vi "Read.vi"(8 "error in (no error)":errorcluster, 11 "CIFTag in":refnum<class "CIFTagI64.lvclass">) -> (0 "error out":errorcluster, 1 "timed out?":bool, 2 "Data":i64, 3 "CIFTag out":refnum<class "CIFTagI64.lvclass">)   [LabVIEW 2021, in "CIFTagI64.lvclass"]
uses:
  CIFTagI64.lvclass
  D:/dev/CIF-LVCore/src/CIFUtilities/CIFChannels/CIFChannels.lvclass
  D:/dev/CIF-LVCore/src/Channels/CIFTag/CIFTag/CIFTag.lvclass
  CIFUtilities/CIFChannels/CIFChannels.lvclass/CIFChannels.ctl
  CIFUtilities/CIFChannels/Typedef/Channel State.ctl
  CIFUtilities/CIFChannels/Typedef/Direction.ctl
  CIFTagI64.lvclass/CIFTagI64.ctl
  CIFTag/CIFTag.lvclass/CIFTag.ctl
  cbead010-ab61-49ec-ac6c-083511305d37.vi
  CIFUtilities/CIFChannels/Accessors/Read Channel State.vi
  CIFUtilities/CIFChannels/Accessors/Read Direction.vi
  CIFUtilities/CIFChannels/Accessors/Write Channel State.vi
  CIFUtilities/CIFChannels/Accessors/Read Disconnect Behavior.vi
  cbead010-ab61-49ec-ac6c-083511305d37.vi/c28b0ead-42ad-4072-80a2-aca7f2bd7ce3.vi
  cbead010-ab61-49ec-ac6c-083511305d37.vi/219d0231-d98b-4193-b5cc-84f90e3c9091.vi
  <vilib>/CIFChannels/SubVIs/Get dll Path.vi
  CIFTag/CIFTag.lvclass
  CIFUtilities/CIFChannels/CIFChannels.lvclass
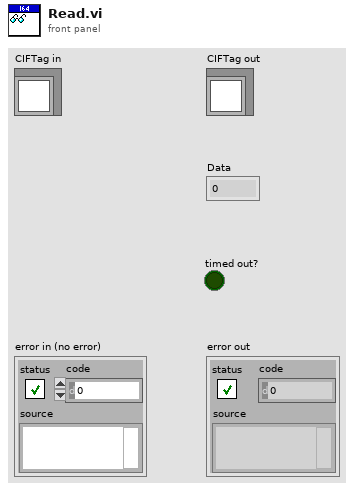
[diagram p1: front panel]
types:
  T1 = typedef "CIFChannels.lvclass/Channel State.ctl" = enum16{"Creating", "Disconnected", "Connecting", "Connected", "Destroying"}
  T2 = typedef "CIFChannels.lvclass/Direction.ctl" = enum16{"Publisher", "Subscriber"}
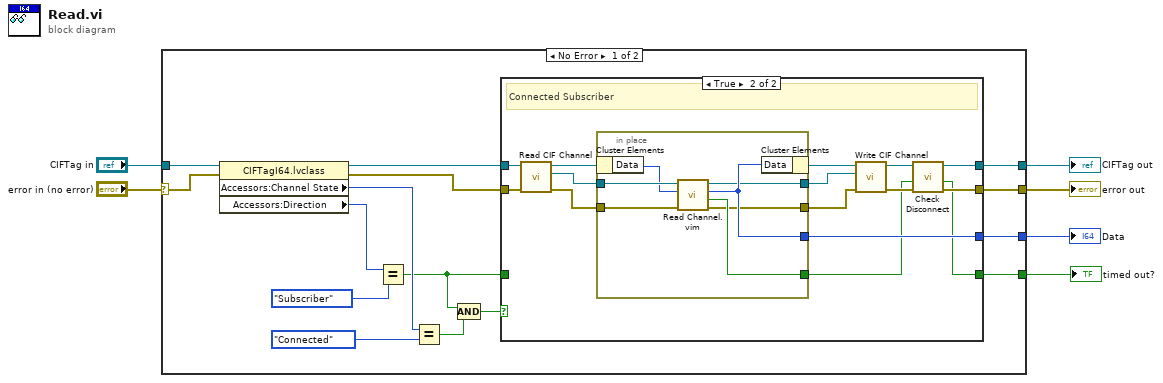
[diagram p0: block diagram]
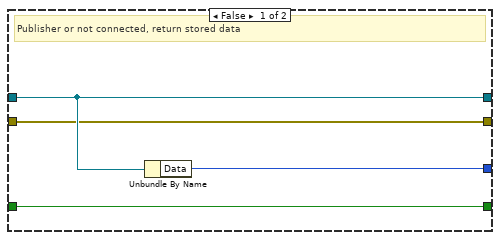
[diagram p2: hidden frame]
diagram:
  n1 = case shown="No Error" "error in (no error)" {
    selector: "error in (no error)" -> [w18 w49]
    tunnel: [w7 w49] -> w5
    tunnel: [w8 w48] -> w3
    tunnel: "CIFTag in" -> [w19 w48]
    tunnel: [w21 _] -> w2
    tunnel: [w20 _] -> w1
    frame No Error {
      n2 = property class="CIFTagI64.lvclass"(reference=w19, error in=w18) -> (reference out=w17:refnum<class "CIFTagI64.lvclass">, error out=w16:errorcluster, "Accessors:Channel State"=w13:T1, "Accessors:Direction"=w15:T2)
      n3 = Equal?(x=w15, y=Direction."Subscriber") -> (x = y?=w9:bool)
      n4 = Equal?(x=w13, y=Channel_State."Connected") -> (x = y?=w11:bool)
      n5 = Compound Arithmetic op=AND(w9, w11) -> (w10:bool)
      n6 = case shown="True" w10 {
        tunnel: [w24 w26] -> w21
        tunnel: [w25 w33] -> w20
        tunnel: w16 -> [w22 w39]
        tunnel: w17 -> [w23 w40]
        tunnel: w9 -> [w24 _]
        tunnel: [w23 w38] -> w8
        tunnel: [w22 w37] -> w7
        frame False {
          # "Publisher or not connected, return stored data"
          n7 = Unbundle By Name(w23) -> ("Data"=w25:i64)
        }
        frame True {
          # "Connected Subscriber"
          n8 = call "Read CIF Channel.vi"("error in (no error)"=w39, "CIFTag in"=w40) -> ("error out"=w34:errorcluster, "CIF Channel"=w35:refnum<k21>, "CIFTag out"=w36:refnum<class "CIFTagI64.lvclass">)  [unwired: 7 in]
          n9 = in-place {
            in-place-border: [w44] -> w27
            in-place-border: w35 -> [w47]
            in-place-border: w34 -> [w45]
            in-place-border: [w43] -> w33
            in-place-border: [w42] -> w30
            in-place-border: [w41] -> w31
            n10 = in-place-cluster #1(w36) -> ("Data"=w46:i64)
            n11 = call "Read Channel.vim"("error in"=w45, "Data in"=w46, "CIF Channel in"=w47) -> ("error out"=w41:errorcluster, "Timed out?"=w44:bool, "Data out"=w43:i64, "CIF Channel out"=w42:refnum<k21>)  [unwired: 5 in]
            n12 = in-place-cluster #1("Data"=w43) -> (w32:refnum<class "CIFTagI64.lvclass">)
          }
          n13 = call "Write CIF Channel.vi"("error in (no error)"=w31, "CIF Channel"=w30, "CIFTag in"=w32) -> ("error out"=w28:errorcluster, "CIFTag out"=w29:refnum<class "CIFTagI64.lvclass">)  [unwired: 7 in]
          n14 = call "Check Disconnect.vi"("error in (no error)"=w28, "timeout in"=w27, "CIFTag in"=w29) -> ("error out"=w37:errorcluster, "timeout out"=w26:bool, "CIFTag out"=w38:refnum<class "CIFTagI64.lvclass">)  [unwired: 5 in, 1 out]
        }
      }
    }
    frame Error {
    }
  }
  "error out" <- w5
  "CIFTag out" <- w3
  "timed out?" <- w2
  "Data" <- w1
